vi "DAQ.initWaveform.vi"(8 "error in (no error)":errorcluster, 11 "DAQ in":refnum<class "DAQ.lvclass">) -> (0 "error out":errorcluster, 2 "Waveforms":waveform(dbl)[](array[waveform]), 3 "DAQ out":refnum<class "DAQ.lvclass">)   [LabVIEW 2016, in "DAQ.lvclass"]
uses:
  DAQ.lvclass
  DAQ.lvclass/DAQ.ctl
  <vilib>/measure/NI_MABase.lvlib
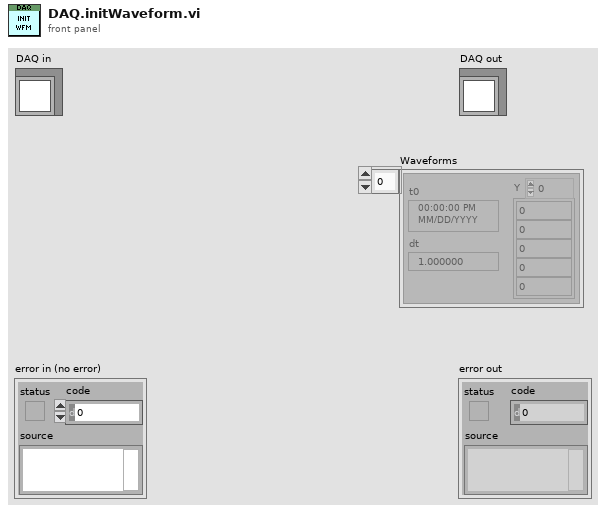
[diagram p1: front panel]
types:
  T1 = typedef "DAQ.lvclass/DAQ_SamplingInfo.ctl" = cluster{"Fs":dbl, "#s":i32}
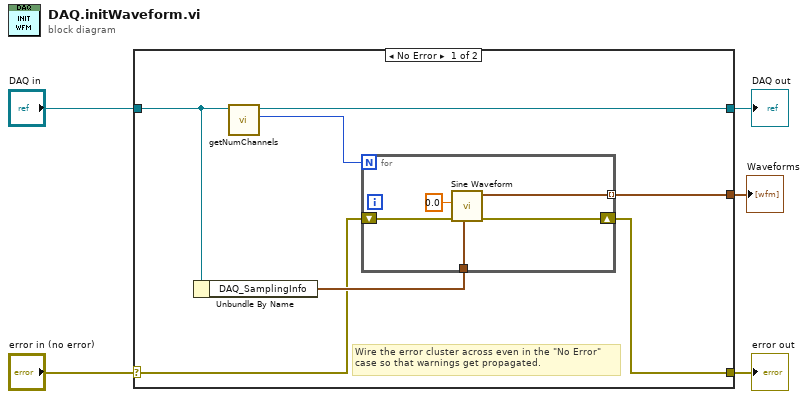
[diagram p0: block diagram]
diagram:
  n1 = case shown="No Error" "error in (no error)" {
    selector: "error in (no error)" -> [w9 w19]
    tunnel: [w10 w19] -> w1
    tunnel: [w7 w18] -> w3
    tunnel: "DAQ in" -> [w8 w18]
    tunnel: [w12 _] -> w2
    frame No Error {
      # "Wire the error cluster across even in the \"No Error\"\ncase so that warnings get propagated."
      n2 = Unbundle By Name(w8) -> ("DAQ_SamplingInfo"=w11:T1)
      n3 = call "getNumChannels.vi"("DAQ in"=w8) -> ("NumChannels"=w6:i32, "DAQ out"=w7:refnum<class "DAQ.lvclass">)  [unwired: 8 in, 1 out]
      n4 = for {
        N: w6 -> [_]
        tunnel: [w17] -> w12 mode=indexing
        tunnel: w11 -> [w16]
        shift-right: [w14] -> w10
        shift-left: w9 -> [w15]
        n5 = call <vilib>:"Sine Waveform.vi"("sampling info"=w16, "error in (no error)"=w15, "amplitude"=0.0) -> ("error out"=w14:errorcluster, "signal out"=w17:waveform(dbl))  [unwired: 7 in]
      }
    }
    frame Error {
    }
  }
  "error out" <- w1
  "DAQ out" <- w3
  "Waveforms" <- w2
